vi "filter_logic.vi"() -> ()   [LabVIEW 2015]
panel:
  in  "constants cluster":T1={"High Charge Limit"=0, "Low Charge Limit"=0, "Low Velocity Count"=0, "High Velocity Count"=0, "Low Velocity Count"=0, 26666666.59375, "High Mass Limit"=0, "Low Mass Limit"=0}
  in  "Filter Specific Constants":T2
  out "Output Cluster":T3
  in  "Variables Cluster":T4
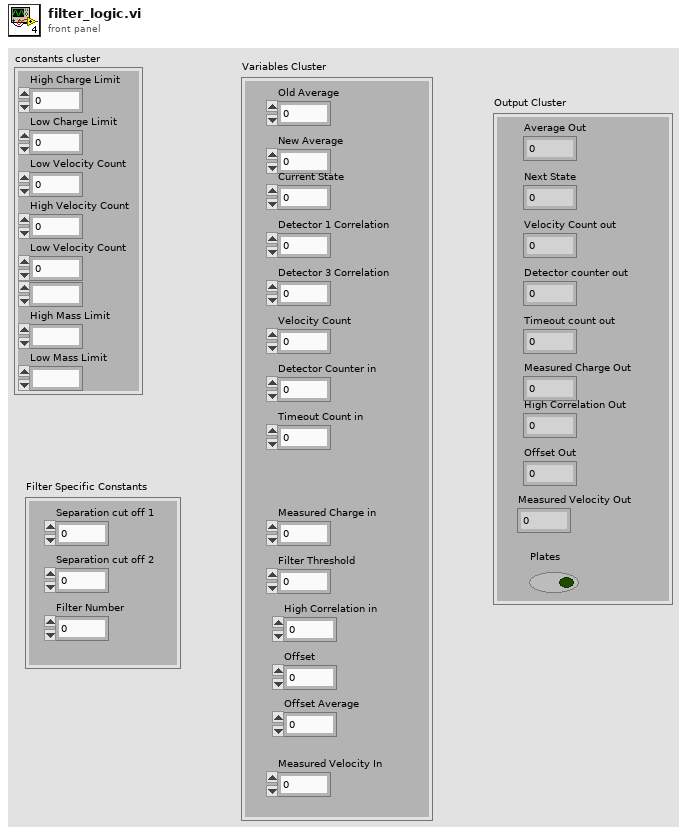
[diagram p1: front panel]
types:
  T1 = cluster{"High Charge Limit":i16, "Low Charge Limit":i16, "Low Velocity Count":i32, "High Velocity Count":i32, "Low Velocity Count":i32, fxp<+,30,25>, "High Mass Limit":i64, "Low Mass Limit":i64}
  T2 = cluster{"Separation cut off 1":i32, "Filter Number":i32, "Separation cut off 2":i32}
  T3 = cluster{"Average Out":i32, "Next State":u8, "Velocity Count out":i32, "Detector counter out":i32, "Timeout count out":u32, "Measured Charge Out":i32, "High Correlation Out":i32, "Plates":bool, "Offset Out":i32, "Measured Velocity Out":i32}
  T4 = cluster{"Old Average":i32, "New Average":i32, "Current State":u8, "Detector 1 Correlation":i32, "Detector 3 Correlation":i32, "Velocity Count":i32, "Detector Counter in":i32, "Timeout Count in":i32, "Measured Charge in":i32, "Filter Threshold":i32, "High Correlation in":i32, "Offset":i32, "Offset Average":i32, "Measured Velocity In":i32}
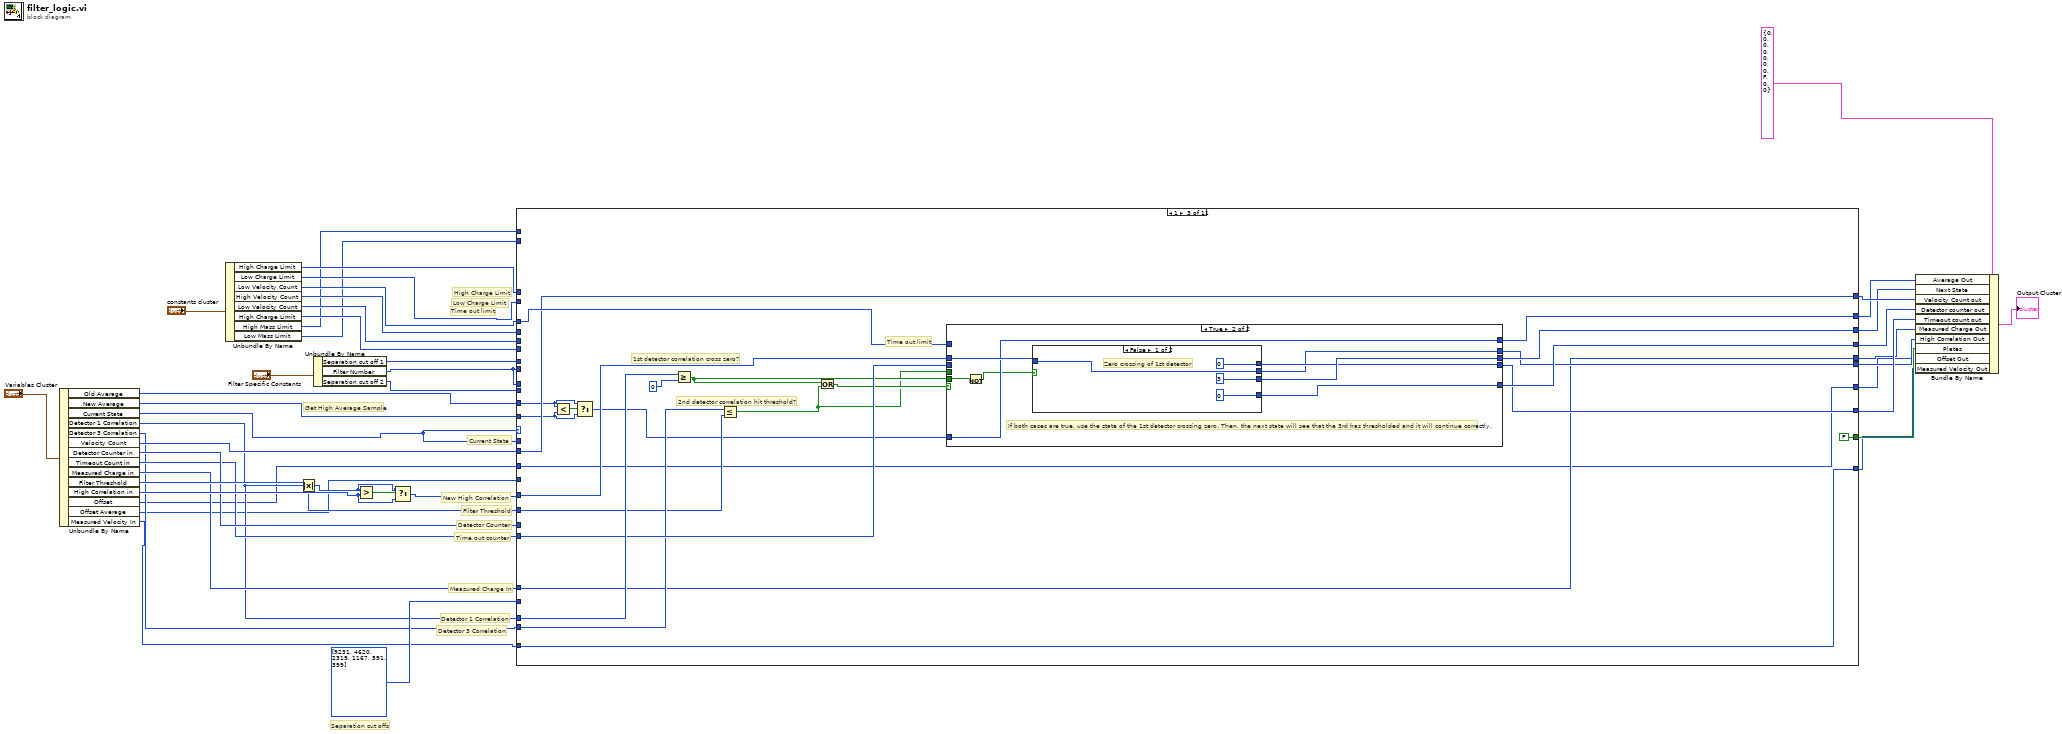
[diagram p0: block diagram]
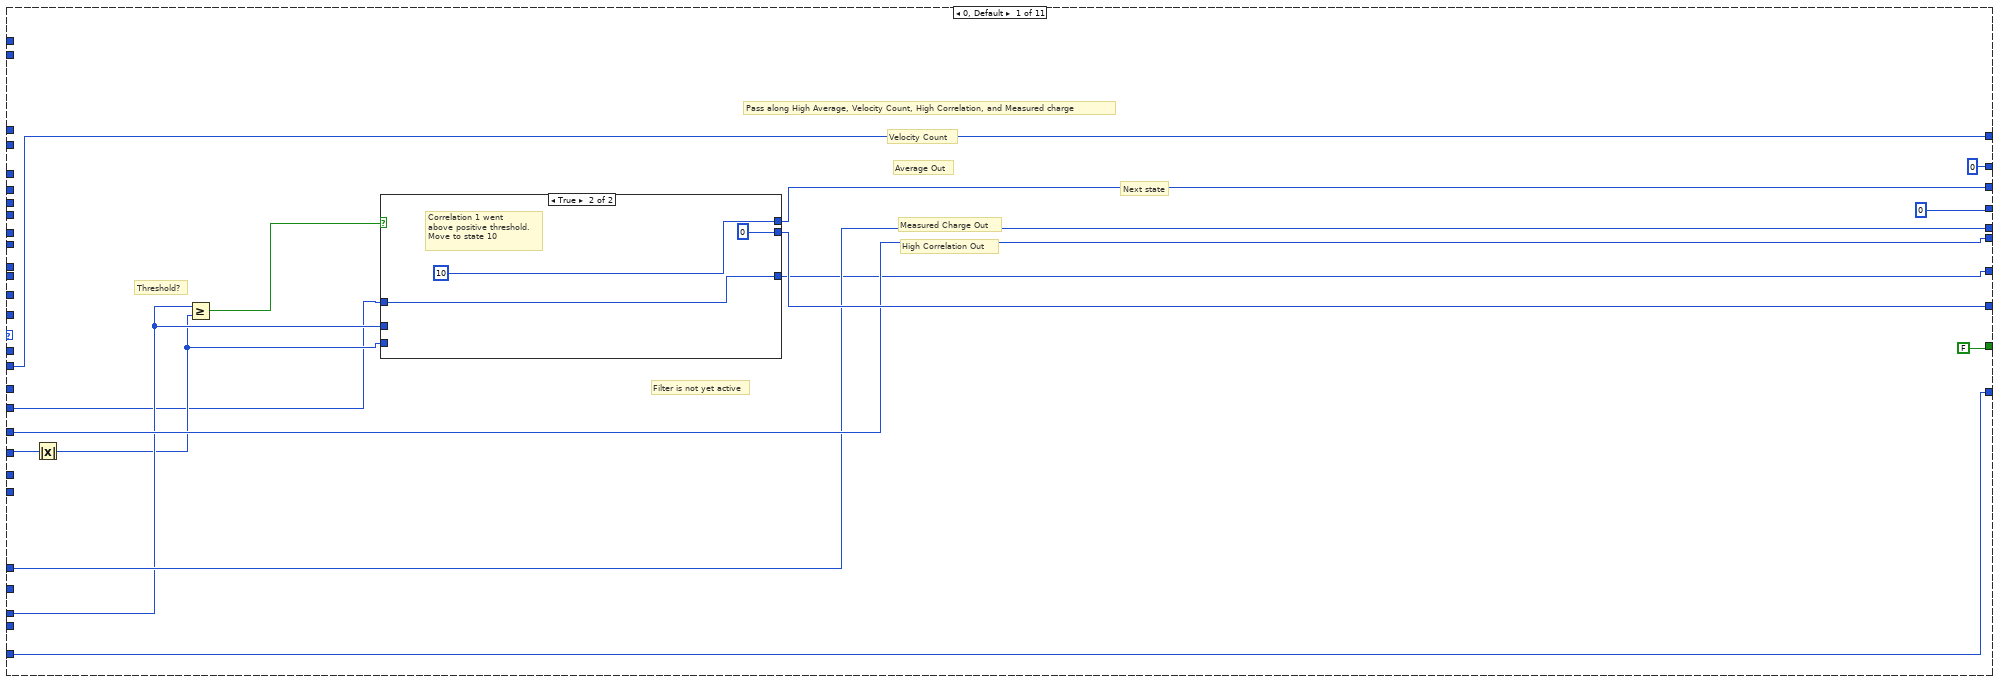
[diagram p2: hidden frame]
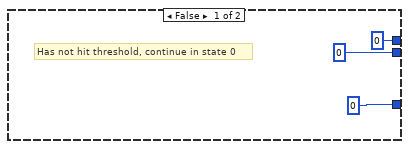
[diagram p3: hidden frame]
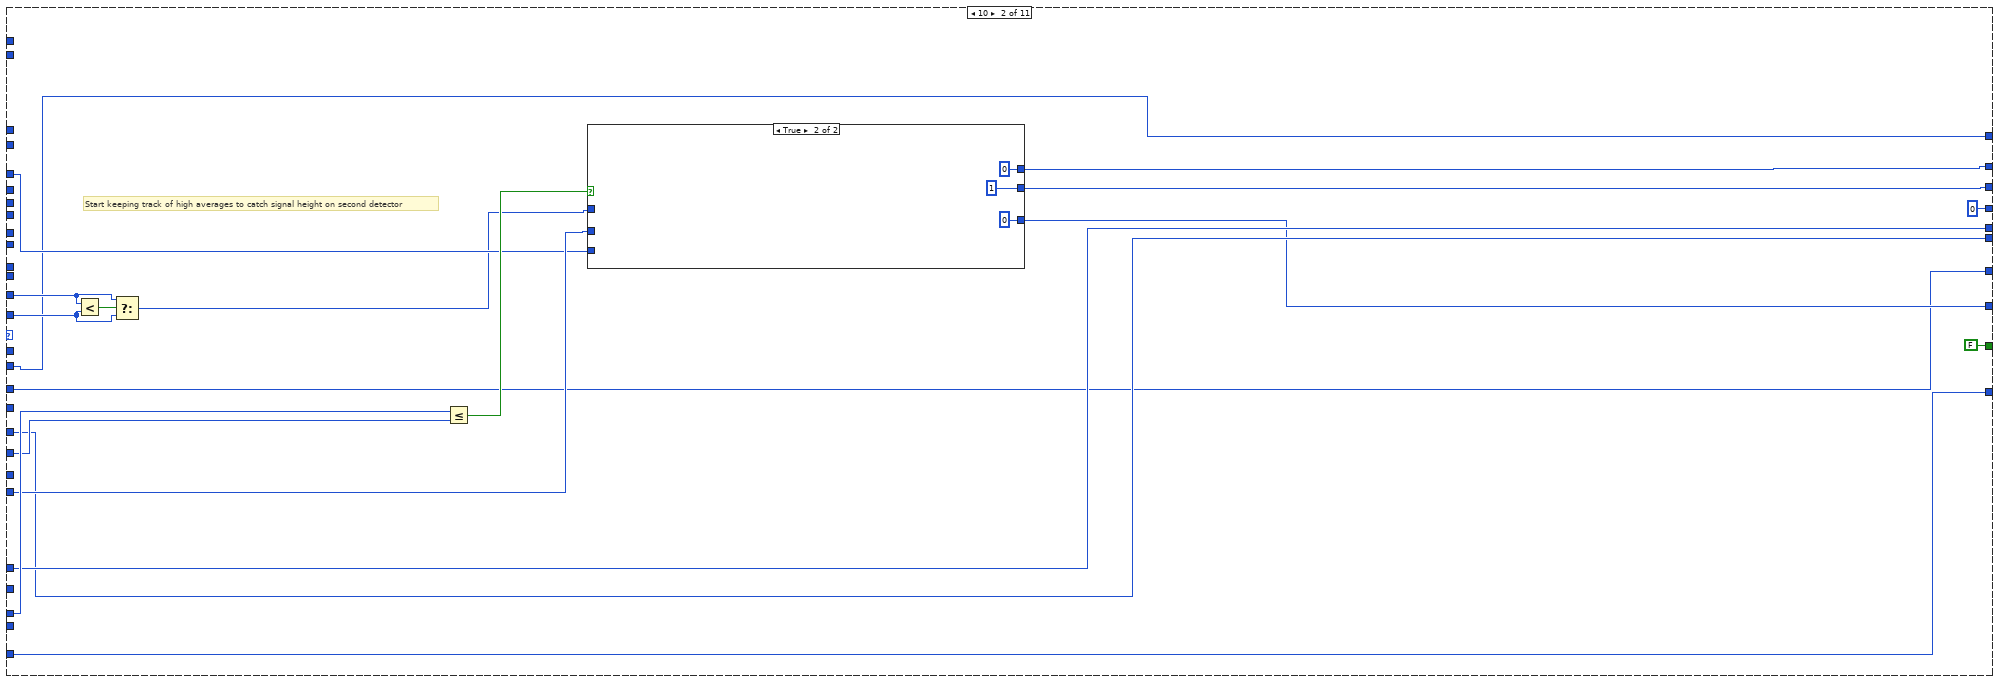
[diagram p4: hidden frame]
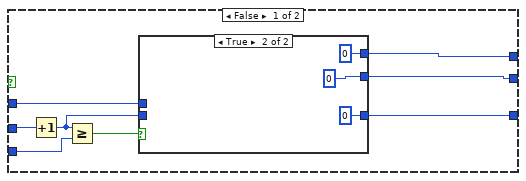
[diagram p5: hidden frame]
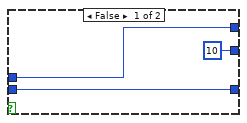
[diagram p6: hidden frame]
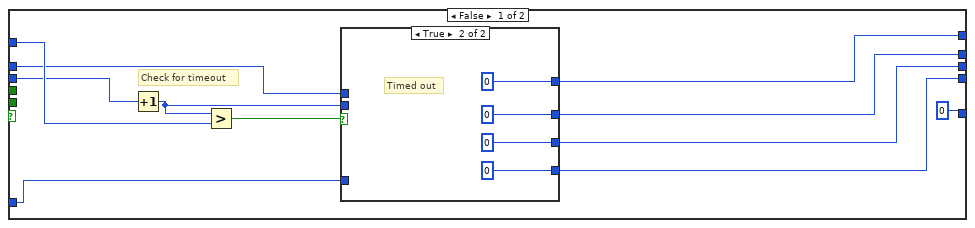
[diagram p7: hidden frame]
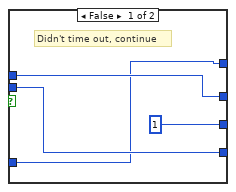
[diagram p8: hidden frame]
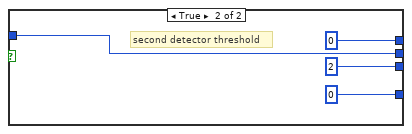
[diagram p9: hidden frame]
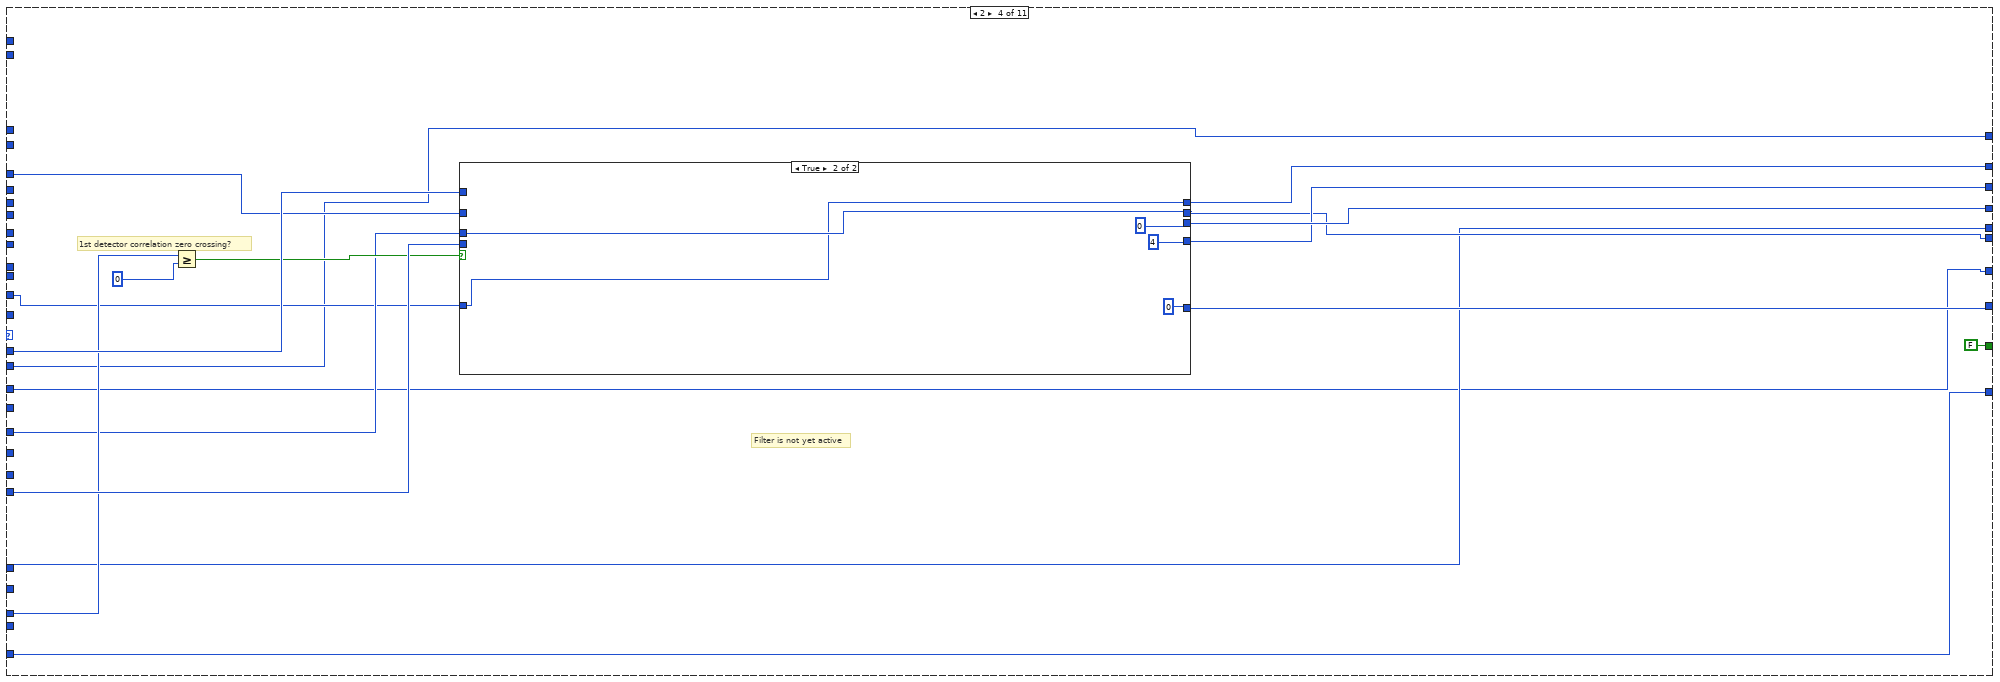
[diagram p10: hidden frame]
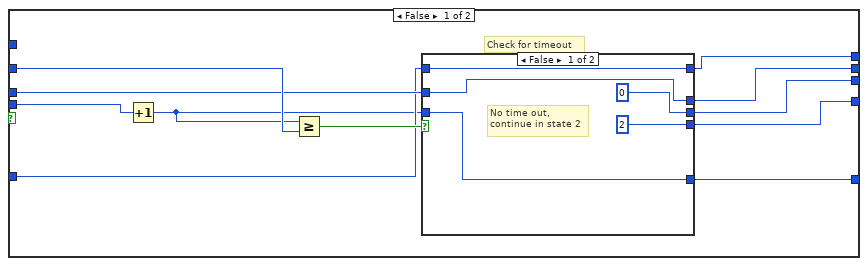
[diagram p11: hidden frame]
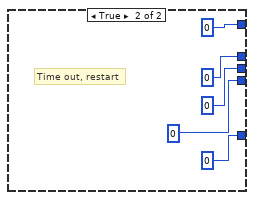
[diagram p12: hidden frame]
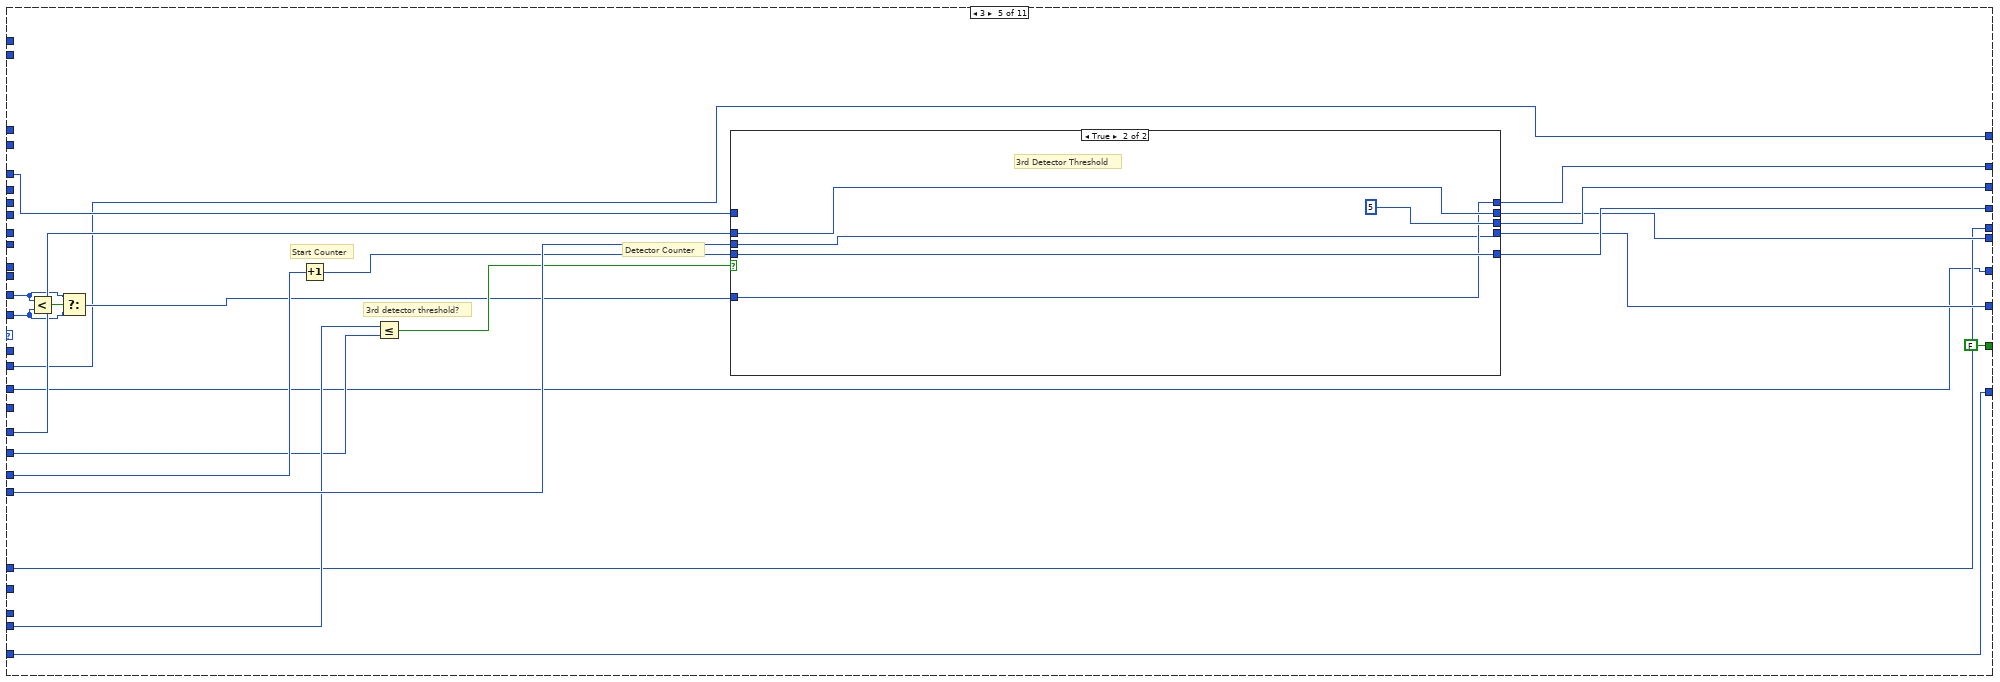
[diagram p13: hidden frame]
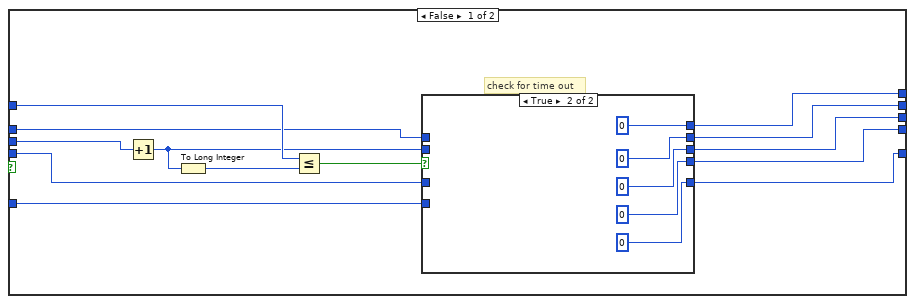
[diagram p14: hidden frame]
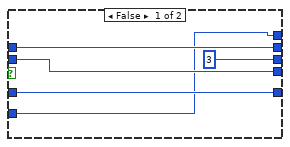
[diagram p15: hidden frame]
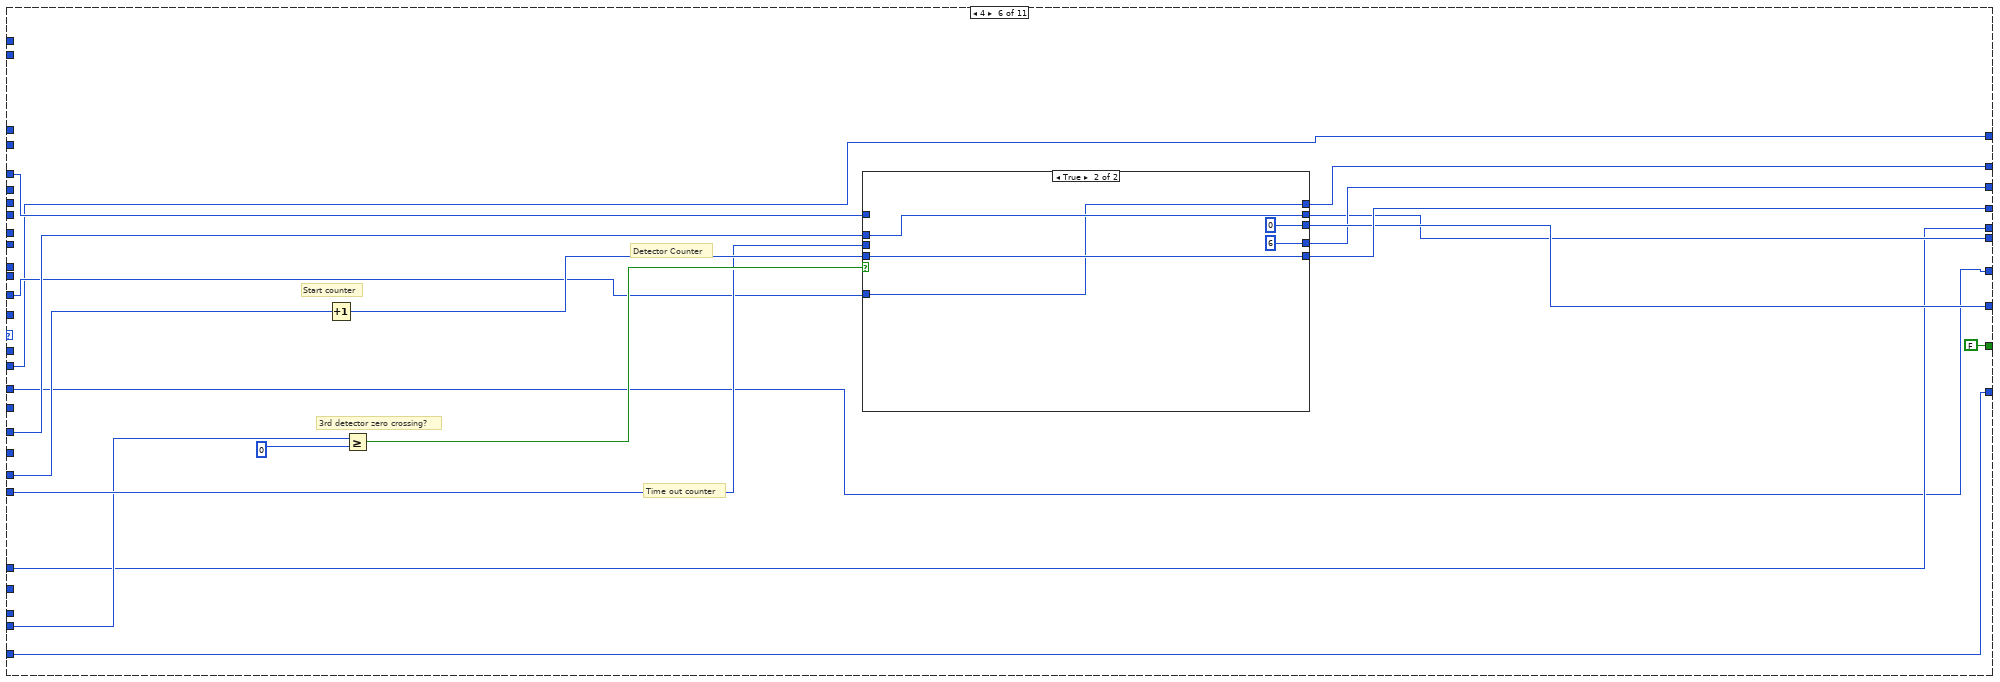
[diagram p16: hidden frame]
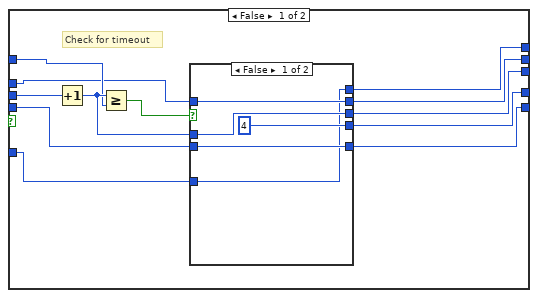
[diagram p17: hidden frame]
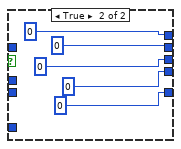
[diagram p18: hidden frame]
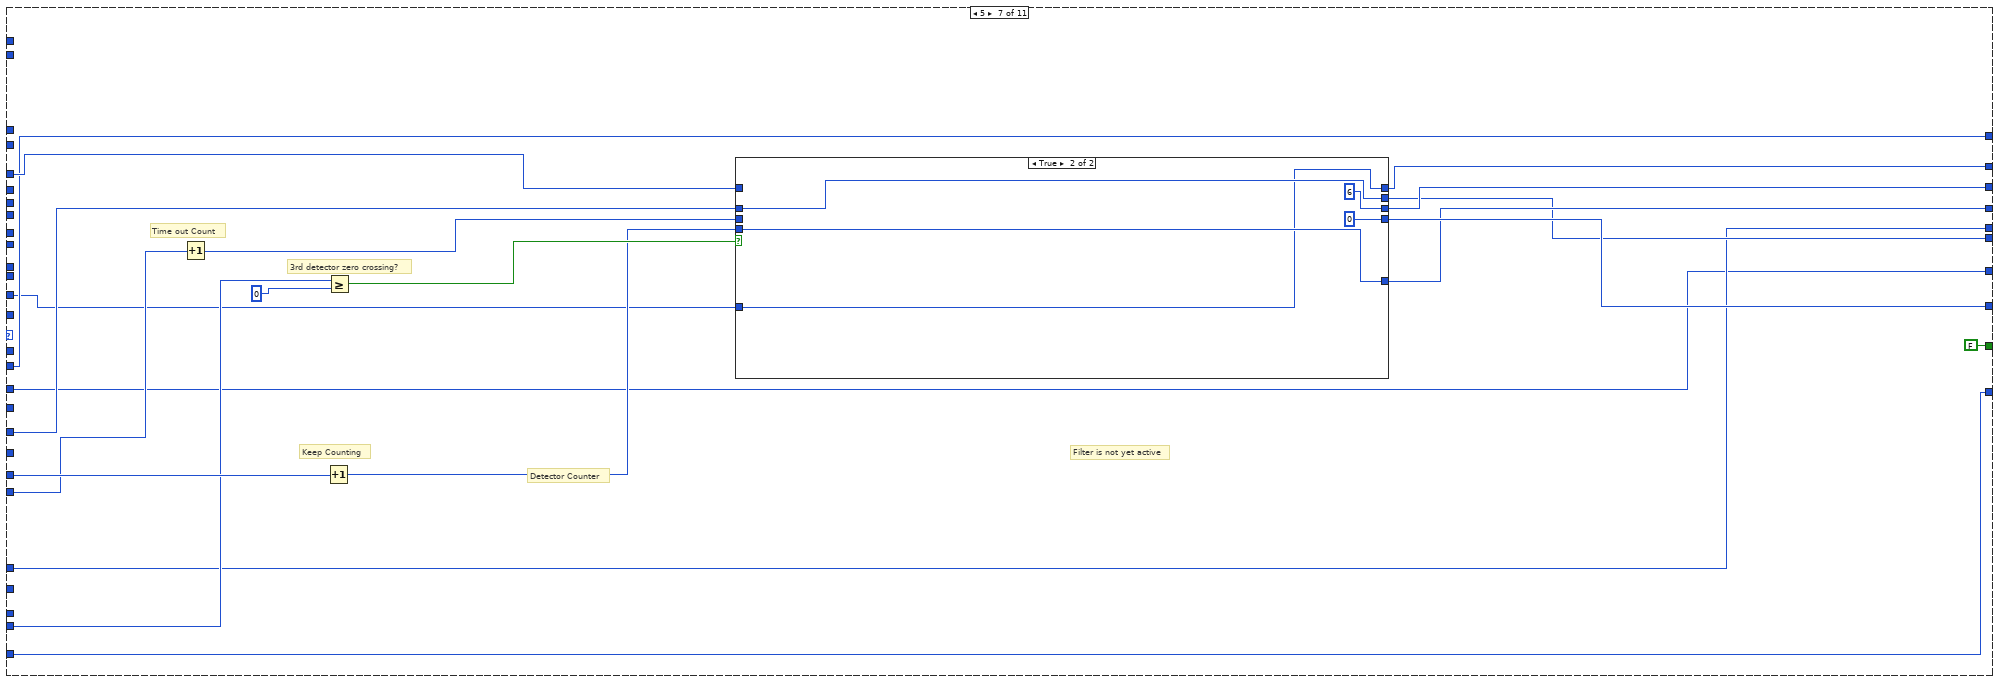
[diagram p19: hidden frame]
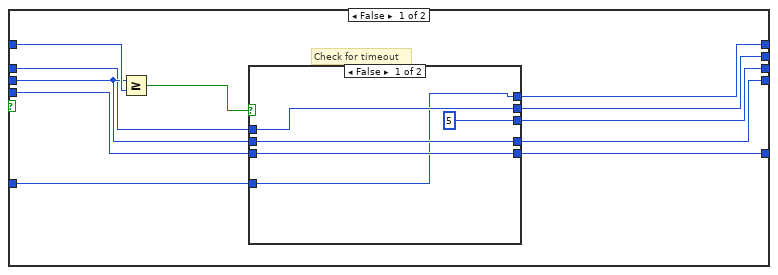
[diagram p20: hidden frame]
diagram:
  # "Detector 3 Correlation"
  # "Detector 1 Correlation"
  # "Separation cut offs"
  # "Measured Charge In"
  # "Time out counter"
  # "Detector Counter"
  # "Filter Threshold"
  # "New High Correlation"
  # "Current State"
  # "Get High Average Sample"
  # "Time out limit"
  # "Low Charge Limit"
  # "High Charge Limit"
  n1 = Unbundle By Name("Variables Cluster") -> ("Old Average"=w17:i32, "New Average"=w16:i32, "Current State"=w38:u8, "Detector 1 Correlation"=w27:i32, "Detector 3 Correlation"=w26:i32, "Velocity Count"=w37:i32, "Detector Counter in"=w31:i32, "Timeout Count in"=w30:i32, "Measured Charge in"=w29:i32, "Filter Threshold"=w32:i32, "High Correlation in"=w33:i32, "Offset"=w15:i32, "Offset Average"=w14:i32, "Measured Velocity In"=w10:i32)
  n2 = Unbundle By Name("constants cluster") -> ("High Charge Limit"=w9:i16, "Low Charge Limit"=w8:i16, "Low Velocity Count"=w7:i32, "High Velocity Count"=w6:i32, "Low Velocity Count"=w5:i32, "High Charge Limit"=w4:i16, "High Mass Limit"=w3:i64, "Low Mass Limit"=w2:i64)
  n3 = Absolute Value(x=w27) -> (abs(x)=w34:i32)
  n4 = Unbundle By Name("Filter Specific Constants") -> ("Separation cut off 1"=w42:i32, "Filter Number"=w41:i32, "Separation cut off 2"=w40:i32)
  n5 = Greater?(x=w34, y=w33) -> (0:w35:bool)
  n6 = Select(t=w34, s=w35, f=w33) -> (s? t:f=w36:i32)
  n7 = case shown="1" w38 {
    tunnel: w27 -> [w51 w81 w125 w172 _ _ _ _ _ _ _]
    tunnel: w26 -> [_ _ w114 _ w218 w265 w310 _ _ _ _]
    tunnel: w32 -> [w49 w80 w113 _ w217 _ _ _ _ _ _]
    tunnel: w31 -> [_ _ _ _ w220 w273 w319 w353 w481 w514 w548]
    tunnel: [0 0 w123 w178 w226 w271 w312 w365 w480 w510 w544] -> w23
    tunnel: [w59 w78 w122 w177 w225 w268 w315 w362 w479 w512 w545] -> w19
    tunnel: w38 -> [_ _ _ w176 _ _ _ _ _ _ _]
    tunnel: w37 -> [w55 w73 w115 w162 w206 w256 w311 w363 w444 w515 w542]
    tunnel: w7 -> [_ w76 w121 w175 w223 w266 w316 _ _ _ _]
    tunnel: w30 -> [_ w77 w120 w174 w224 w267 w318 _ w468 _ _]
    tunnel: [w58 w68 w119 w173 w222 w269 w314 u32 0 w467 u32 0 ("Timeout Count in") u32 0] -> w22
    tunnel: w5 -> [_ _ _ _ _ _ _ _ w478 _ _]
    tunnel: w6 -> [_ _ _ _ _ _ _ _ w477 _ _]
    tunnel: [w55 w73 w115 w162 w206 w256 w311 w364 w476 w511 w542] -> w25
    tunnel: i32[] [9231, 4620, 2319, 1167, 591, 399] -> [_ _ _ _ _ _ _ w356 _ _ _]
    tunnel: w8 -> [_ _ _ _ _ _ _ _ w475 _ _]
    tunnel: w9 -> [_ _ _ _ _ _ _ _ w474 _ _]
    tunnel: w36 -> [w54 w70 w112 w169 w216 w259 w308 w360 w473 w508 w540]
    tunnel: [w54 w70 w111 w168 w215 w263 w307 w361 w472 w508 w541] -> w20
    tunnel: w29 -> [w53 w71 w110 w167 w214 w262 w306 w359 w471 w503 w536]
    tunnel: [w53 w71 w110 w167 w214 w262 w306 w359 w470 w504 w536] -> w21
    tunnel: [0 ("Old Average In") w74 w109 w166 w213 w261 w305 w358 w458 w500 0 ("Old Average In")] -> w24
    tunnel: w42 -> [_ _ _ _ _ _ _ w355 _ _ _]
    tunnel: w41 -> [_ _ _ _ _ _ _ w357 _ _ _]
    tunnel: w41 -> [_ _ _ _ _ _ _ w351 w469 w513 w539]
    tunnel: w40 -> [_ _ _ _ _ _ _ w354 _ _ _]
    tunnel: [FALSE FALSE ("Data") FALSE FALSE FALSE FALSE FALSE FALSE w464 w507 w535] -> w18
    tunnel: w17 -> [_ w83 w106 w164 w210 w258 w303 w349 w458 w500 _]
    tunnel: w16 -> [_ w82 w105 _ w209 _ _ _ _ _ _]
    tunnel: w15 -> [_ w67 w103 w163 w207 w257 w302 w348 w459 w499 _]
    tunnel: w14 -> [w46 _ _ _ _ _ _ _ _ _ _]
    tunnel: [w47 w67 w103 w163 w207 w257 w302 w348 w459 w499 0 ("Offset")] -> w13
    tunnel: [w45 w66 w102 w161 w205 w255 w301 w347 w461 w505 w533] -> w11
    tunnel: w10 -> [w45 w66 w102 w161 w205 w255 w301 w347 w460 w506 w533]
    tunnel: w4 -> [_ _ _ _ _ _ _ _ _ _ _]
    tunnel: w3 -> [_ _ _ _ _ _ _ _ w457 _ _]
    tunnel: w2 -> [_ _ _ _ _ _ _ _ w456 _ _]
    frame 0, Default {
      # "Filter is not yet active"
      # "High Correlation Out"
      # "Measured Charge Out"
      # "Next state"
      # "Average Out"
      # "Velocity Count"
      # "Pass along High Average, Velocity Count, High Correlation, and Measured charge"
      # "Threshold?"
      n8 = Absolute Value(x=w49) -> (abs(x)=w48:i32)
      n9 = Greater Or Equal?(x=w51, y=w48) -> (x >= y?=w56:bool)
      n10 = case shown="True" w56 {
        tunnel: [u8 0 u8 10] -> w59
        tunnel: [u32 0 u32 0] -> w58
        tunnel: w51 -> [_ _]
        tunnel: w48 -> [_ _]
        tunnel: [0 w63] -> w47
        tunnel: w46 -> [_ w63]
        frame False {
          # "Has not hit threshold, continue in state 0"
        }
        frame True {
          # "Correlation 1 went\nabove positive threshold.\nMove to state 10"
        }
      }
    }
    frame 10 {
      # "Start keeping track of high averages to catch signal height on second detector"
      n11 = Less?(x=w83, y=w82) -> (x < y?=w84:bool)
      n12 = Select(t=w83, s=w84, f=w82) -> (s? t:f=w75:i32)
      n13 = Less Or Equal?(x=w81, y=w80) -> (x <= y?=w79:bool)
      n14 = case shown="True" w79 {
        tunnel: [w90 u8 1] -> w78
        tunnel: w77 -> [w87 _]
        tunnel: w76 -> [w92 _]
        tunnel: w75 -> [w89 _]
        tunnel: [w88 0 ("New Average")] -> w74
        tunnel: [w85 0] -> w68
        frame False {
          n15 = Increment(x=w87) -> (x+1=w86:i32)
          n16 = Greater Or Equal?(x=w86, y=w92) -> (x >= y?=w91:bool)
          n17 = case shown="True" w91 {
            tunnel: [u8 10 u8 0] -> w90
            tunnel: w89 -> [w95 _]
            tunnel: [w95 0 ("New Average")] -> w88
            tunnel: w86 -> [w93 _]
            tunnel: [w93 0] -> w85
            frame False {
            }
            frame True {
            }
          }
        }
        frame True {
        }
      }
    }
    frame 1 {
      # "Time out limit"
      # "2nd detector correlation hit threshold?"
      # "1st detector correlation cross zero?"
      n18 = Less?(x=w106, y=w105) -> (x < y?=w107:bool)
      n19 = Select(t=w106, s=w107, f=w105) -> (s? t:f=w104:i32)
      n20 = Greater Or Equal?(x=w125, y=0) -> (x >= y?=w117:bool)
      n21 = Less Or Equal?(x=w114, y=w113) -> (x <= y?=w116:bool)
      n22 = Or(x=w117, y=w116) -> (x .or. y?=w118:bool)
      n23 = case shown="True" w118 {
        tunnel: [0 w151] -> w123
        tunnel: [w134 w152] -> w122
        tunnel: w121 -> [w136 _]
        tunnel: w120 -> [w133 _]
        tunnel: [w132 w150] -> w119
        tunnel: w117 -> [_ w146]
        tunnel: w116 -> [_ _]
        tunnel: w112 -> [w130 w149]
        tunnel: [w129 w148] -> w111
        tunnel: [w128 w147] -> w109
        tunnel: w104 -> [w126 w147]
        frame False {
          # "Check for timeout"
          n24 = Increment(x=w133) -> (x+1=w127:i32)
          n25 = Greater?(x=w127, y=w136) -> (0:w135:bool)
          n26 = case shown="True" w135 {
            tunnel: [u8 1 u8 0] -> w134
            tunnel: w127 -> [w139 _]
            tunnel: [w139 u32 0] -> w132
            tunnel: w130 -> [w138 _]
            tunnel: [w138 0 ("High Correlation In")] -> w129
            tunnel: [w137 0 ("Old Average In")] -> w128
            tunnel: w126 -> [w137 _]
            frame False {
              # "Didn't time out, continue"
            }
            frame True {
              # "Timed out"
            }
          }
        }
        frame True {
          # "If both cases are true, use the state of the 1st detector crossing zero. Then, the next state will see that the 3rd has thresholded and it will continue correctly."
          n27 = Not(x=w146) -> (.not. x?=w145:bool)
          n28 = case shown="False" w145 {
            tunnel: [u8 3 u8 2] -> w152
            tunnel: [0 0] -> w151
            tunnel: [u32 0 u32 0] -> w150
            tunnel: w149 -> [w153 w157]
            tunnel: [w153 w157] -> w148
            frame False {
              # "Zero crossing of 1st detector"
            }
            frame True {
              # "second detector threshold"
            }
          }
        }
      }
    }
    frame 2 {
      # "Filter is not yet active"
      # "1st detector correlation zero crossing?"
      n29 = Greater Or Equal?(x=w172, y=0) -> (x >= y?=w170:bool)
      n30 = case shown="True" w170 {
        tunnel: [w184 0] -> w178
        tunnel: [w188 u8 4] -> w177
        tunnel: w176 -> [_ _]
        tunnel: w175 -> [w187 _]
        tunnel: w174 -> [w185 _]
        tunnel: [w186 u32 0] -> w173
        tunnel: w169 -> [w183 w201]
        tunnel: [w182 w201] -> w168
        tunnel: [w181 w200] -> w166
        tunnel: w164 -> [w180 w200]
        frame False {
          # "Check for timeout"
          n31 = Increment(x=w185) -> (x+1=w179:i32)
          n32 = Greater Or Equal?(x=w179, y=w187) -> (x >= y?=w189:bool)
          n33 = case shown="False" w189 {
            tunnel: [u8 2 u8 0] -> w188
            tunnel: w179 -> [w194 _]
            tunnel: [w194 u32 0] -> w186
            tunnel: [0 0] -> w184
            tunnel: w183 -> [w191 _]
            tunnel: [w191 0 ("High Correlation In")] -> w182
            tunnel: [w190 0 ("Old Average In")] -> w181
            tunnel: w180 -> [w190 _]
            frame False {
              # "No time out, \ncontinue in state 2"
            }
            frame True {
              # "Time out, restart"
            }
          }
        }
        frame True {
        }
      }
    }
    frame 3 {
      # "3rd detector threshold?"
      # "Start Counter"
      # "Detector Counter"
      n34 = Less?(x=w210, y=w209) -> (x < y?=w211:bool)
      n35 = Select(t=w210, s=w211, f=w209) -> (s? t:f=w208:i32)
      n36 = Increment(x=w220) -> (x+1=w219:i32)
      n37 = Less Or Equal?(x=w218, y=w217) -> (x <= y?=w221:bool)
      n38 = case shown="True" w221 {
        tunnel: w219 -> [w234 w254]
        tunnel: [w233 w254] -> w226
        tunnel: [w236 u8 5] -> w225
        tunnel: w224 -> [w232 w250]
        tunnel: w223 -> [w239 _]
        tunnel: [w235 w250] -> w222
        tunnel: w216 -> [w230 w252]
        tunnel: [w229 w252] -> w215
        tunnel: [w228 w251] -> w213
        tunnel: w208 -> [w227 w251]
        frame False {
          # "check for time out"
          n39 = Increment(x=w232) -> (x+1=w231:i32)
          n40 = To Long Integer(number=w231) -> (32bit integer=w238:i32)
          n41 = Less Or Equal?(x=w239, y=w238) -> (x <= y?=w237:bool)
          n42 = case shown="True" w237 {
            tunnel: [u8 3 u8 0] -> w236
            tunnel: w231 -> [w243 _]
            tunnel: [w243 u32 0] -> w235
            tunnel: w234 -> [w242 _]
            tunnel: [w242 0] -> w233
            tunnel: w230 -> [w241 _]
            tunnel: [w241 0 ("High Correlation In")] -> w229
            tunnel: [w240 0 ("Old Average In")] -> w228
            tunnel: w227 -> [w240 _]
            frame False {
            }
            frame True {
            }
          }
        }
        frame True {
          # "3rd Detector Threshold"
        }
      }
    }
    frame 4 {
      # "Time out counter"
      # "3rd detector zero crossing?"
      # "Start counter"
      # "Detector Counter"
      n43 = Increment(x=w273) -> (x+1=w270:i32)
      n44 = Greater Or Equal?(x=w265, y=0) -> (x >= y?=w272:bool)
      n45 = case shown="True" w272 {
        tunnel: [w278 w300] -> w271
        tunnel: w270 -> [w279 w300]
        tunnel: [w281 u32 0] -> w269
        tunnel: [w283 u8 6] -> w268
        tunnel: w267 -> [w285 _]
        tunnel: w266 -> [w280 _]
        tunnel: w259 -> [w277 w297]
        tunnel: [w276 w297] -> w263
        tunnel: [w275 w296] -> w261
        tunnel: w258 -> [w274 w296]
        frame False {
          # "Check for timeout"
          n46 = Increment(x=w285) -> (x+1=w282:i32)
          n47 = Greater Or Equal?(x=w282, y=w280) -> (x >= y?=w284:bool)
          n48 = case shown="False" w284 {
            tunnel: [u8 4 u8 0] -> w283
            tunnel: w282 -> [w289 _]
            tunnel: [w289 u32 0] -> w281
            tunnel: w279 -> [w288 _]
            tunnel: [w288 0] -> w278
            tunnel: w277 -> [w287 _]
            tunnel: [w287 0 ("High Correlation In")] -> w276
            tunnel: [w286 0 ("Old Average In")] -> w275
            tunnel: w274 -> [w286 _]
            frame False {
            }
            frame True {
            }
          }
        }
        frame True {
        }
      }
    }
    frame 5 {
      # "Filter is not yet active"
      # "Time out Count"
      # "3rd detector zero crossing?"
      # "Keep Counting"
      # "Detector Counter"
      n49 = Increment(x=w318) -> (x+1=w317:i32)
      n50 = Increment(x=w319) -> (x+1=w313:i32)
      n51 = Greater Or Equal?(x=w310, y=0) -> (x >= y?=w320:bool)
      n52 = case shown="True" w320 {
        tunnel: w317 -> [w327 _]
        tunnel: w316 -> [w331 _]
        tunnel: [w329 u8 6] -> w315
        tunnel: [w328 u32 0] -> w314
        tunnel: w313 -> [w326 w344]
        tunnel: [w325 w344] -> w312
        tunnel: w308 -> [w323 w343]
        tunnel: [w324 w343] -> w307
        tunnel: [w322 w342] -> w305
        tunnel: w303 -> [w321 w342]
        frame False {
          # "Check for timeout"
          n53 = Greater Or Equal?(x=w327, y=w331) -> (x >= y?=w330:bool)
          n54 = case shown="False" w330 {
            tunnel: [u8 5 u8 0] -> w329
            tunnel: [w335 u32 0] -> w328
            tunnel: w327 -> [w335 _]
            tunnel: w326 -> [w334 _]
            tunnel: [w334 0] -> w325
            tunnel: [w333 0 ("High Correlation In")] -> w324
            tunnel: w323 -> [w333 _]
            tunnel: [w332 0 ("Old Average In")] -> w322
            tunnel: w321 -> [w332 _]
            frame False {
            }
            frame True {
            }
          }
        }
        frame True {
        }
      }
    }
    frame 6 {
      # "Does the velocity of this particle most closely match this filter?"
      # "Detector Counter"
      n55 = case shown="4" w351 {
        tunnel: w356 -> [w374 w380 w384 w393 w403 w411 w420 w430]
        tunnel: w355 -> [w373 w379 w383 w392 w401 w410 w419 w429]
        tunnel: w354 -> [w372 _ w385 w394 w402 w412 w421 _]
        tunnel: w353 -> [w370 w378 w382 w391 w400 w409 w418 w427]
        tunnel: [w369 w376 w381 w390 w399 w408 w417 w426] -> w352
        frame 0, Default {
          n56 = Index Array(array=w374, index=w373) -> (element=w371:i32)
          n57 = Index Array(array=w374, index=w372) -> (element=w375:i32)
          n58 = Greater Or Equal?(x=w370, y=w375) -> (x >= y?=w368:bool)
          n59 = Less?(x=w370, y=w371) -> (x < y?=w367:bool)
          n60 = And(x=w368, y=w367) -> (x .and. y?=w369:bool)
        }
        frame 1 {
          n61 = Index Array(array=w380, index=w379) -> (element=w377:i32)
          n62 = Greater Or Equal?(x=w378, y=w377) -> (x >= y?=w376:bool)
        }
        frame 2 {
          n63 = Index Array(array=w384, index=w383) -> (element=w387:i32)
          n64 = Index Array(array=w384, index=w385) -> (element=w386:i32)
          n65 = Greater Or Equal?(x=w382, y=w386) -> (x >= y?=w388:bool)
          n66 = Less?(x=w382, y=w387) -> (x < y?=w389:bool)
          n67 = And(x=w388, y=w389) -> (x .and. y?=w381:bool)
        }
        frame 3 {
          n68 = Index Array(array=w393, index=w392) -> (element=w396:i32)
          n69 = Index Array(array=w393, index=w394) -> (element=w395:i32)
          n70 = Greater Or Equal?(x=w391, y=w395) -> (x >= y?=w397:bool)
          n71 = Less?(x=w391, y=w396) -> (x < y?=w398:bool)
          n72 = And(x=w397, y=w398) -> (x .and. y?=w390:bool)
        }
        frame 4 {
          # "3"
          # "2"
          n73 = Index Array(array=w403, index=w401) -> (element=w405:i32)
          n74 = Index Array(array=w403, index=w402) -> (element=w404:i32)
          n75 = Greater Or Equal?(x=w400, y=w404) -> (x >= y?=w406:bool)
          n76 = Less?(x=w400, y=w405) -> (x < y?=w407:bool)
          n77 = And(x=w406, y=w407) -> (x .and. y?=w399:bool)
        }
        frame 5 {
          n78 = Index Array(array=w411, index=w410) -> (element=w414:i32)
          n79 = Index Array(array=w411, index=w412) -> (element=w413:i32)
          n80 = Greater Or Equal?(x=w409, y=w413) -> (x >= y?=w415:bool)
          n81 = Less?(x=w409, y=w414) -> (x < y?=w416:bool)
          n82 = And(x=w415, y=w416) -> (x .and. y?=w408:bool)
        }
        frame 6 {
          n83 = Index Array(array=w420, index=w419) -> (element=w424:i32)
          n84 = Index Array(array=w420, index=w421) -> (element=w425:i32)
          n85 = Greater Or Equal?(x=w418, y=w425) -> (x >= y?=w423:bool)
          n86 = Less?(x=w418, y=w424) -> (x < y?=w422:bool)
          n87 = And(x=w423, y=w422) -> (x .and. y?=w417:bool)
        }
        frame 7 {
          n88 = Index Array(array=w430, index=w429) -> (element=w428:i32)
          n89 = Less?(x=w427, y=w428) -> (x < y?=w426:bool)
        }
      }
      n90 = case shown="True" w352 {
        tunnel: [0 w441] -> w365
        tunnel: w353 -> [_ w440]
        tunnel: [w435 w440] -> w364
        tunnel: w363 -> [w435 _]
        tunnel: [u8 0 u8 7] -> w362
        tunnel: [0 ("High Correlation In") w438] -> w361
        tunnel: w360 -> [_ w438]
        tunnel: [0 ("Old Average In") w437] -> w358
        tunnel: w357 -> [_ _]
        tunnel: w349 -> [_ w437]
        frame False {
          # "Incorrect filter, restart"
        }
        frame True {
          (unwired) fxp<+,31,3> 7.340293329209089
          # "Use this number for 3rd detector"
          # "Filter is now active"
          # "Number of cycles to wait until\nopening the plates"
          # "This is applying a multiplier, which is derived from the ratio of lengths of\ndet3 to deflection plates vs. det1 to det3. It includes 15 cm\nof slop, as well as -1.666 detector length, since a signal that is perfectly\nmatched to a filter will have its second zero crossing 1 and 2/3 detector \nlength away from the edge of the 3rd detector"
          # "Correct filter\nCalculate \"wait\" number of cycles"
          n91 = To Fixed-Point(number=w440) -> (fixed-point=w443:fxp<+/-,32,32>)  [unwired: 1 in]
          n92 = Multiply(x=w443, y=fxp<+,22,1> 1.636110782623291) -> (x*y=w442:fxp<+/-,54,33>)
          n93 = To Long Integer(number=w442) -> (32bit integer=w441:i32)
        }
      }
    }
    frame 7 {
      # "Did the particle meet the mass conditions?"
      # "calculated mass of particle"
      # "Get charge from smoothed data"
      # "Check Velocity Conditions"
      # "Check Charge Conditions"
      # "Detector Counter"
      n94 = Subtract(x=w459, y=w458) -> (x-y=w463:i32)
      n95 = Square(x=w444) -> (x^2=w448:i32)
      n96 = To Quad Integer(1:w448) -> (0:w447:i64)
      n97 = Absolute Value(x=w463) -> (abs(x)=w445:i32)
      n98 = To Quad Integer(1:w445) -> (0:w446:i64)
      n99 = Multiply(x=w447, y=w446) -> (x*y=w449:i64)
      n100 = Less Or Equal?(x=w449, y=w457) -> (x <= y?=w450:bool)
      n101 = Greater Or Equal?(x=w449, y=w456) -> (x >= y?=w451:bool)
      n102 = Greater Or Equal?(x=w444, y=w477) -> (x >= y?=w452:bool)
      n103 = Less Or Equal?(x=w444, y=w478) -> (x <= y?=w453:bool)
      n104 = To Word Integer(number=w445) -> (16bit integer=w466:i16)
      n105 = To Word Integer(number=w445) -> (16bit integer=w465:i16)
      n106 = Less Or Equal?(x=w475, y=w466) -> (x <= y?=w454:bool)
      n107 = Greater Or Equal?(x=w474, y=w465) -> (x >= y?=w455:bool)
      n108 = Compound Arithmetic op=AND(w450, w451, w452, w453, w454, w455) -> (w462:bool)
      n109 = case shown="True" w462 {
        tunnel: w481 -> [_ w498]
        tunnel: w444 -> [w488 w492]
        tunnel: [0 w496] -> w480
        tunnel: [u8 0 u8 8] -> w479
        tunnel: [w488 w492] -> w476
        tunnel: w473 -> [_ w497]
        tunnel: [0 ("High Correlation In") w497] -> w472
        tunnel: w471 -> [w485 w490]
        tunnel: w445 -> [_ _]
        tunnel: [w485 w490] -> w470
        tunnel: w469 -> [_ _]
        tunnel: w468 -> [_ _]
        tunnel: [u32 0 ("Timeout Count in") 0 ("Timeout Count in")] -> w467
        tunnel: [FALSE ("Data") FALSE ("Data")] -> w464
        tunnel: [w482 w491] -> w461
        tunnel: w460 -> [w482 w491]
        frame False {
          # "Correct filter, but wrong velocity and/or charge."
          # "Did not meet conditions, restart"
        }
        frame True {
          # "Met Conditions"
          # "Count \"Detector Counter\" down"
          n110 = Decrement(x=w498) -> (x-1=w496:i32)
        }
      }
    }
    frame 8 {
      # "Met Conditions, declare that this filter is active and count down until opening the plates"
      # "Count \"Detector Counter\" down"
      # "velocity count"
      n111 = Subtract(x=w499, y=w500) -> (x-y=w502:i32)
      n112 = Absolute Value(x=w502) -> (abs(x)=w501:i32)
      n113 = Decrement(x=w514) -> (x-1=w516:i32)
      n114 = Less Or Equal?(x=w516, y=0) -> (x <= y?=w517:bool)
      n115 = case shown="True" w517 {
        tunnel: [u8 8 u8 9] -> w512
        tunnel: [w524 w531] -> w510
        tunnel: w515 -> [w522 w526]
        tunnel: w516 -> [w524 _]
        tunnel: [w522 w526] -> w511
        tunnel: w513 -> [_ _]
        tunnel: [FALSE ("Data") TRUE ("Data")] -> w507
        tunnel: w506 -> [w520 _]
        tunnel: [w520 w526] -> w505
        tunnel: [w519 w525] -> w504
        tunnel: w503 -> [w519 _]
        tunnel: w501 -> [_ w525]
        frame False {
          # "Counting down to wait to open the plates"
        }
        frame True {
          # "Plates are available so\nallow access to plates"
          # "velocity count"
          # "Number derived from ratio of lengths of plates (w/ 25cm of slop)\n vs. det1 to det3"
          # "clock counts to wait \nuntil close."
          # "Need to open the plates\nhere. Check availablility of plates, and if available, set memory to true to open them"
          n116 = To Fixed-Point(number=w526) -> (fixed-point=w528:fxp<+/-,32,32>)  [unwired: 1 in]
          n117 = Multiply(x=w528, y=fxp<+,18,0> 0.7666587829589844 ("x")) -> (x*y=w532:fxp<+/-,50,32>)
          n118 = To Long Integer(number=w532) -> (32bit integer=w531:i32)
        }
      }
    }
    frame 9 {
      # "Count down and then close plates"
      # "Detector Counter"
      n119 = Decrement(x=w548) -> (x-1=w543:i32)
      n120 = Less Or Equal?(x=w543, y=0) -> (x <= y?=w546:bool)
      n121 = case shown="True" w546 {
        tunnel: [w551 0] -> w544
        tunnel: [u8 9 u8 0] -> w545
        tunnel: w543 -> [w551 _]
        tunnel: w540 -> [w550 _]
        tunnel: [w550 0 ("Noise Level")] -> w541
        tunnel: w539 -> [_ _]
        tunnel: [TRUE ("Data") FALSE ("Data")] -> w535
        frame False {
          # "Count down to wait to close the plates"
        }
        frame True {
          # "Restart"
          # "Close plates here"
        }
      }
    }
  }
  n122 = Bundle By Name(cluster=T3 {"Average Out"=0, "Next State"=0, "Velocity Count out"=0, "Detector counter out"=0, "Timeout count out"=0, "Measured Charge Out"=0, "High Correlation Out"=0, "Plates"=FALSE, "Offset Out"=0, "Measured Velocity Out"=0} ("Output Cluster"), "Average Out"=w24, "Next State"=w19, "Velocity Count out"=w25, "Detector counter out"=w23, "Timeout count out"=w22, "Measured Charge Out"=w21, "High Correlation Out"=w20, "Plates"=w18, "Offset Out"=w13, "Measured Velocity Out"=w11) -> (→"Output Cluster":T3)
